vi "Autonomous Independent.vi"() -> ()   [LabVIEW 2023]
doc: "This VI is called when autonomous begins, and will automatically be terminated when autonomous ends. You can carry out timed or sensor driven robot movement independently without needing to return to the caller."
uses:
  <vilib>/Rock Robotics/WPI/SafetyOutput/WPI_SafetyOutputConfigMenu.ctl
  <vilib>/Rock Robotics/WPI/RobotDrive/WPI_RobotDriveDevRef.ctl
  <vilib>/Rock Robotics/WPI/MotorControl/WPI_MotorControlDeviceRef.ctl
  <vilib>/Rock Robotics/WPI/MotorControl/WPI_MotorControlType.ctl
  <vilib>/Rock Robotics/SystemInterfaces/DIO/FPGA_DIOPWMChannel.ctl
  <vilib>/Rock Robotics/WPI/PWM/WPI_PWMDeadband.ctl
  <vilib>/Rock Robotics/SystemInterfaces/DIO/FPGA_DIOChannel.ctl
  <vilib>/Rock Robotics/WPI/ThirdParty/REV Robotics/REVLib/Typedef/Spark MAX Idle Mode.ctl
  <vilib>/Rock Robotics/WPI/Utilities/WPI_GetSetVariantRefNum.vi
  <vilib>/Rock Robotics/Network Tables/NT Read String.vi
  <vilib>/Rock Robotics/Network Tables/NT Write Numeric Array.vi
  <vilib>/Rock Robotics/WPI/ThirdParty/REV Robotics/REVLib/SubVI/Public/SPARK Open Brushed.vi
  <vilib>/Rock Robotics/WPI/ThirdParty/REV Robotics/REVLib/SubVI/Public/SPARK Configure Basic Idle Mode.vi
  <vilib>/Rock Robotics/WPI/ThirdParty/REV Robotics/REVLib/SubVI/Public/SPARK Configure Power Smart Current Limit.vi
  <vilib>/Rock Robotics/WPI/RobotDrive/WPI_RobotDriveArcadeDrive_Standard(NoSaturation).vi
panel:
  out "Current Movement, for debugging":T1 {"Y Joystick Value" scale=1.0..-1.0; "X Joystick Value" scale=-1.0..1.0}
  in  "Array of robot movements":T2(array[cluster])=[{"X Joystick Value"=0.39393939393939403, "Y Joystick Value"=0.0, "Delay (sec)"=1.0, "Movement Name"="turn"}, {"X Joystick Value"=-0.3737373737373737, "Y Joystick Value"=0.0, "Delay (sec)"=1.0, "Movement Name"="turn back"}] {"Y Joystick Value" scale=1.0..-1.0; "X Joystick Value" scale=-1.0..1.0}
  # "Be sure to right-click and choose Data Operations>>Make Current Value default if you want to save the array values with the VI"
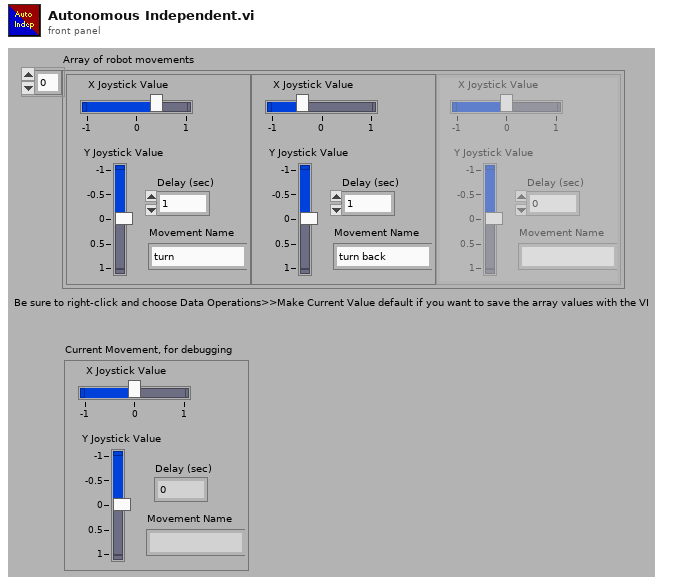
[diagram p1: front panel]
types:
  T1 = cluster{"X Joystick Value":dbl, "Y Joystick Value":dbl, "Delay (sec)":dbl, "Movement Name":string}
  T2 = cluster{"X Joystick Value":dbl, "Y Joystick Value":dbl, "Delay (sec)":dbl, "Movement Name":string}[]
  T3 = typedef "WPI_RobotDriveDevRef.ctl" = cluster{"DevStatus":errorcluster, "Motors[]":T4[], "Square Inputs":bool, "Max Output":dbl}
  T4 = typedef "WPI_MotorControlDeviceRef.ctl" = cluster{"DeviceStatus":errorcluster, "Type":T5, "PWM":cluster{"PWM Channel":T6, "DeadBand":T7}, "CAN":cluster{"Device Number":u8, "SetOutput VI Ref":variant, "GetOutput VI Ref":variant, "Enable VI Ref":variant, "Disable VI Ref":variant, "Data":variant}, "Invert":bool, "DIO PWM":cluster{"PWM \"Enable\" Channel":T6, "DIOChannel":T8, "PWM Rate":dbl}}
  T5 = typedef "WPI_MotorControlType.ctl" = enum16{"PWM", "CAN", "DIO PWM"}
  T6 = typedef "FPGA_DIOPWMChannel.ctl" = enum8{"PWM 0", "PWM 1", "PWM 2", "PWM 3", "PWM 4", "PWM 5", "PWM 6", "PWM 7", "PWM 8", "PWM 9", "PWM MXP 0", "PWM MXP 1", "PWM MXP 2", "PWM MXP 3", "PWM MXP 4", "PWM MXP 5", "PWM MXP 6", "PWM MXP 7", "PWM MXP 8", "PWM MXP 9", "Invalid"}
  T7 = typedef "WPI_PWMDeadband.ctl" = cluster{"Name":string, "maxPositivePwm":i32, "minPositivePwm":i32, "centerPwm":i32, "maxNegativePwm":i32, "minNegativePwm":i32, "angularRange":u16}
  T8 = typedef "FPGA_DIOChannel.ctl" = enum8{"DIO 0", "DIO 1", "DIO 2", "DIO 3", "DIO 4", "DIO 5", "DIO 6", "DIO 7", "DIO 8", "DIO 9", "DIO MXP 0", "DIO MXP 1", "DIO MXP 2", "DIO MXP 3", "DIO MXP 4", "DIO MXP 5", "DIO MXP 6", "DIO MXP 7", "DIO MXP 8", "DIO MXP 9", "DIO MXP 10", "DIO MXP 11", "DIO MXP 12", "DIO MXP 13", "DIO MXP 14", "DIO MXP 15", "SPI Port CS1", "SPI Port CS2", "SPI Port CS3", "SPI Port MISO", "SPI Port MOSI", "Invalid"}
  T9 = typedef "WPI_SafetyOutputConfigMenu.ctl" = enum16{"Enable", "Disable"}
  T10 = typedef "WPI_JoystickDevRef.ctl" = cluster{"Device":T11}
  T11 = typedef "WPI_JoystickDeviceEnum.ctl" = enum16{"USB 0", "USB 1", "USB 2", "USB 3", "USB 4", "USB 5"}
  T12 = typedef "Spark MAX Idle Mode.ctl" = enum16{"Coast", "Brake"}
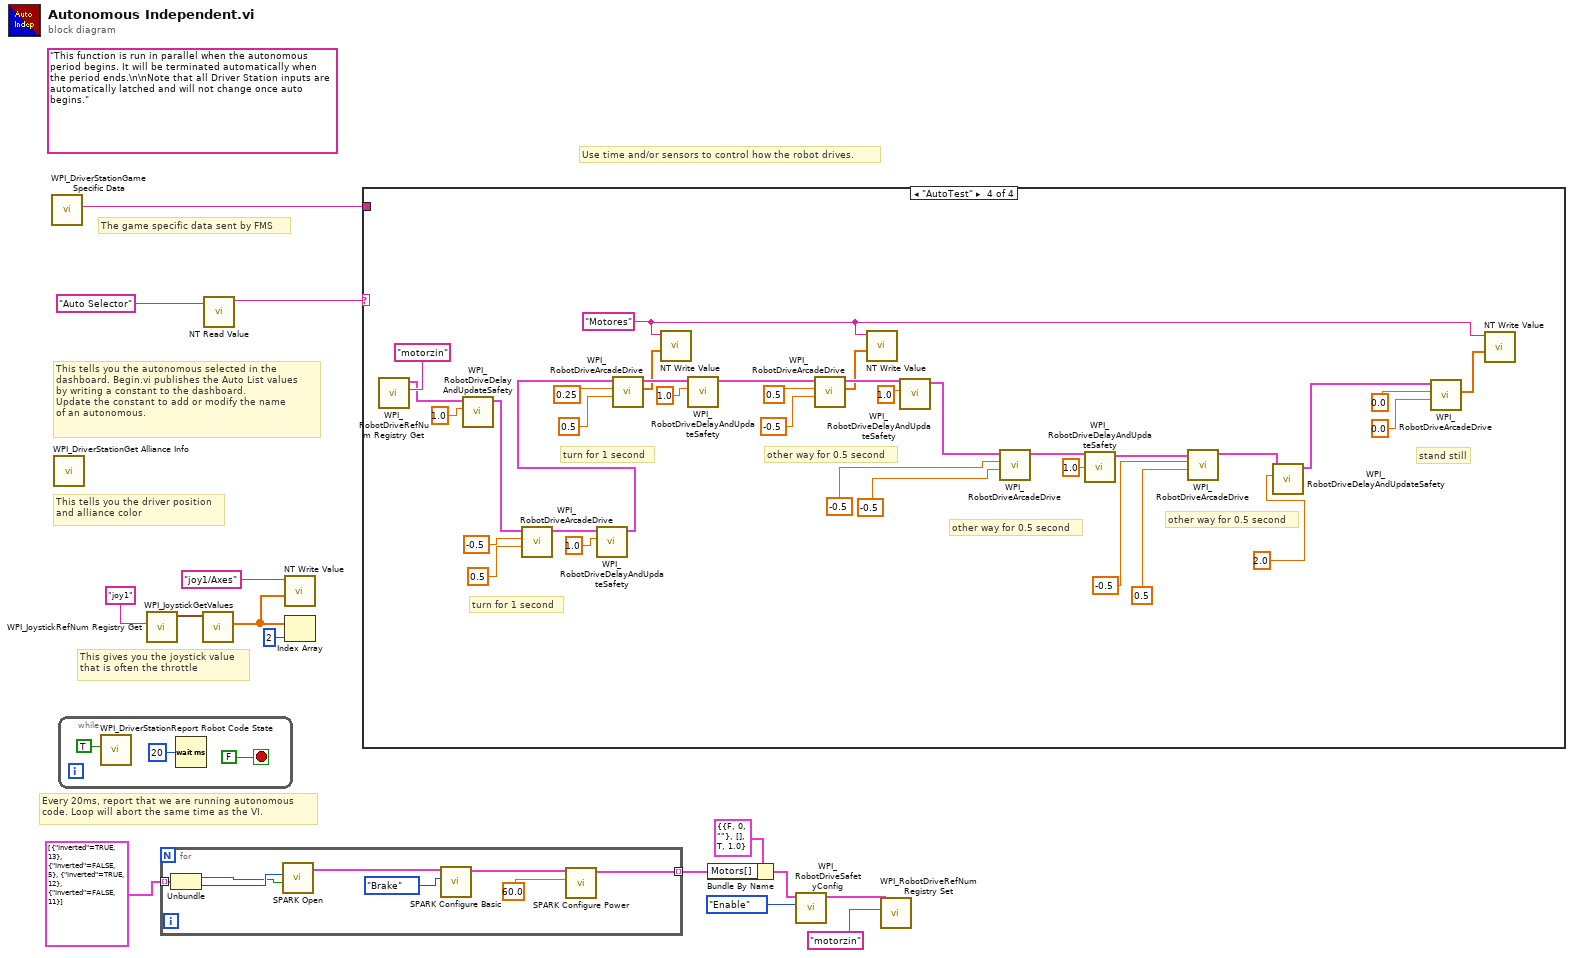
[diagram p0: block diagram]
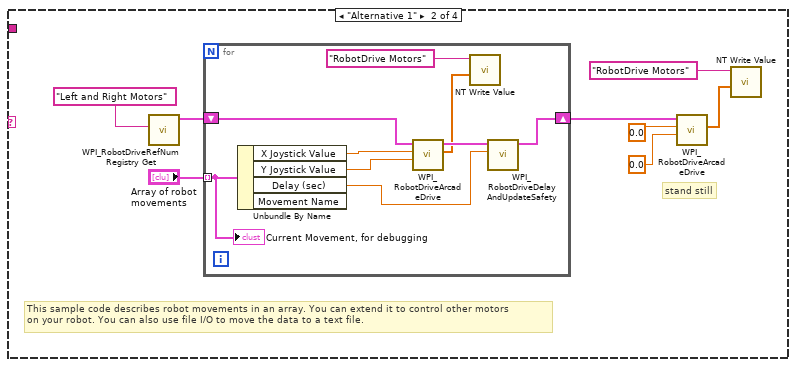
[diagram p3: hidden frame]
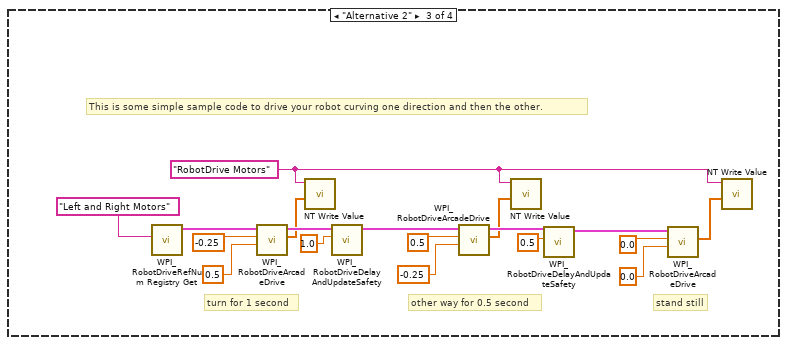
[diagram p4: hidden frame]
diagram:
  (unwired) "This function is run in parallel when the autonomous period begins. It will be terminated automatically when the period ends.\n\nNote that all Driver Station inputs are automatically latched and will not change once auto begins."
  # "The game specific data sent by FMS"
  # "This tells you the autonomous selected in the \ndashboard. Begin.vi publishes the Auto List values\nby writing a constant to the dashboard.\nUpdate the constant to add or modify the name\nof an autonomous."
  # "Every 20ms, report that we are running autonomous\ncode. Loop will abort the same time as the VI."
  # "This gives you the joystick value\nthat is often the throttle"
  # "Use time and/or sensors to control how the robot drives."
  # "This tells you the driver position\nand alliance color"
  n1 = call <vilib>:"WPI_DriverStationGame Specific Data.vi"() -> ("Game Specific Data"=w8:string)  [unwired: 11 in]
  n2 = call <vilib>:"WPI_DriverStationGet Alliance Info.vi"() -> ()  [unwired: 12 out]
  n3 = while {
    stop <- FALSE stop-if-true
    n4 = call <vilib>:"WPI_DriverStationReport Robot Code State.vi"("Autonomous"=TRUE) -> ()  [unwired: 10 in, 1 out]
    n5 = Wait (ms)(milliseconds to wait=u32 20) -> ()  [unwired: 1 out]
  }
  n6 = call <vilib>:"WPI_JoystickRefNum Registry Get.vi"("refnum name"="joy1") -> ("JoystickDevRef"=w14:T10)  [unwired: 1 in, 9 out]
  n7 = for {
    tunnel: cluster{"Inverted":bool, i32}[] [{"Inverted"=TRUE, 13}, {"Inverted"=FALSE, 5}, {"Inverted"=TRUE, 12}, {"Inverted"=FALSE, 11}] ("Array") -> [w26] mode=indexing
    tunnel: [w19] -> w3 mode=indexing
    n8 = Unbundle(w26) -> ("Inverted"=w24:bool, w25:i32)
    n9 = call-poly <vilib>:"SPARK Open.vi"("Invert"=w24, "Device Number"=w25) -> ("MotorControlDeviceRef"=w23:T4)  [unwired: 8 in, 1 out]
    n10 = call-poly <vilib>:"SPARK Configure Basic.vi"("Idle Mode"=Spark_MAX_Idle_Mode."Brake", "MotorControlDeviceRef in"=w23) -> ("MotorControlDeviceRef out"=w22:T4)  [unwired: 8 in, 1 out]
    n11 = call-poly <vilib>:"SPARK Configure Power.vi"("Primay Current Limit (80A)"=60.0, "MotorControlDeviceRef in"=w22) -> ("MotorControlDeviceRef out"=w19:T4)  [unwired: 8 in, 1 out]
  }
  n12 = call <vilib>:"WPI_JoystickGetValues.vi"("JoystickDevRef"=w14) -> ("Axes"=w10:dbl[])  [unwired: 6 in, 4 out]
  n13 = call-poly <vilib>:"NT Read Value.vi"("name"="Auto Selector" ("Name")) -> ("value"=w11:string)  [unwired: 8 in, 2 out]
  n14 = call-poly <vilib>:"NT Write Value.vi"("value"=w10, "name"="joy1/Axes" ("Name")) -> ()  [unwired: 9 in, 1 out]
  n15 = Index Array(array=w10, index=2) -> ()  [unwired: 1 out]
  n16 = case shown="\"AutoTest\"" w11 {
    tunnel: w8 -> [_ _ _ _]
    frame Default {
      # "You can put your main auto here, or you can right-click on the case and make any\nother frame be the default case."
      # "This is the frame that will execute if no selection is made, or if it is not recognized"
    }
    frame "Alternative 1" {
      # "stand still"
      # "This sample code describes robot movements in an array. You can extend it to control other motors\non your robot. You can also use file I/O to move the data to a text file."
      n17 = call <vilib>:"WPI_RobotDriveRefNum Registry Get.vi"("refnum name"="Left and Right Motors") -> ("RobotDriveDevRef"=w33:T3)  [unwired: 1 in, 9 out]
      n18 = for {
        shift-right: [w41] -> w28
        shift-left: w33 -> [w42]
        tunnel: "Array of robot movements" -> [w37] mode=indexing
        n19 = Unbundle By Name(w37) -> ("X Joystick Value"=w40:dbl, "Y Joystick Value"=w39:dbl, "Delay (sec)"=w38:dbl)  [unwired: 1 out]
        n20 = call-poly <vilib>:"WPI_RobotDriveArcadeDrive.vi"("Y axis value"=w39, "X axis value"=w40, "RobotDriveDevRef"=w42) -> ("Motor Values"=w35:dbl[], "RobotDriveDevRef"=w43:T3)  [unwired: 1 in, 6 out]
        n21 = call-poly <vilib>:"NT Write Value.vi"("value"=w35, "name"="RobotDrive Motors" ("Name")) -> ()  [unwired: 9 in, 1 out]
        n22 = call <vilib>:"WPI_RobotDriveDelayAndUpdateSafety.vi"("Delay (s)"=w38, "RobotDriveDevRef"=w43) -> ("RobotDriveDevRef 2"=w41:T3)  [unwired: 8 in, 1 out]
        "Current Movement, for debugging" <- w37
      }
      n23 = call-poly <vilib>:"WPI_RobotDriveArcadeDrive.vi"("Y axis value"=0.0 ("X axis value"), "X axis value"=0.0, "RobotDriveDevRef"=w28) -> ("Motor Values"=w31:dbl[])  [unwired: 1 in, 7 out]
      n24 = call-poly <vilib>:"NT Write Value.vi"("value"=w31, "name"="RobotDrive Motors" ("Name")) -> ()  [unwired: 9 in, 1 out]
    }
    frame "Alternative 2" {
      w45 = "RobotDrive Motors" ("Name")
      # "This is some simple sample code to drive your robot curving one direction and then the other."
      # "stand still"
      # "other way for 0.5 second"
      # "turn for 1 second"
      n25 = call <vilib>:"WPI_RobotDriveRefNum Registry Get.vi"("refnum name"="Left and Right Motors") -> ("RobotDriveDevRef"=w61:T3)  [unwired: 1 in, 9 out]
      n26 = call-poly <vilib>:"WPI_RobotDriveArcadeDrive.vi"("Y axis value"=0.5 ("X axis value"), "X axis value"=-0.25, "RobotDriveDevRef"=w61) -> ("Motor Values"=w44:dbl[], "RobotDriveDevRef"=w54:T3)  [unwired: 1 in, 6 out]
      n27 = call-poly <vilib>:"NT Write Value.vi"("value"=w44, "name"=w45) -> ()  [unwired: 9 in, 1 out]
      n28 = call <vilib>:"WPI_RobotDriveDelayAndUpdateSafety.vi"("Delay (s)"=1.0, "RobotDriveDevRef"=w54) -> ("RobotDriveDevRef 2"=w55:T3)  [unwired: 8 in, 1 out]
      n29 = call-poly <vilib>:"WPI_RobotDriveArcadeDrive.vi"("Y axis value"=-0.25 ("X axis value"), "X axis value"=0.5, "RobotDriveDevRef"=w55) -> ("Motor Values"=w46:dbl[], "RobotDriveDevRef"=w56:T3)  [unwired: 1 in, 6 out]
      n30 = call-poly <vilib>:"NT Write Value.vi"("value"=w46, "name"=w45) -> ()  [unwired: 9 in, 1 out]
      n31 = call <vilib>:"WPI_RobotDriveDelayAndUpdateSafety.vi"("Delay (s)"=0.5, "RobotDriveDevRef"=w56) -> ("RobotDriveDevRef 2"=w57:T3)  [unwired: 8 in, 1 out]
      n32 = call-poly <vilib>:"WPI_RobotDriveArcadeDrive.vi"("Y axis value"=0.0 ("X axis value"), "X axis value"=0.0, "RobotDriveDevRef"=w57) -> ("Motor Values"=w47:dbl[])  [unwired: 1 in, 7 out]
      n33 = call-poly <vilib>:"NT Write Value.vi"("value"=w47, "name"=w45) -> ()  [unwired: 9 in, 1 out]
    }
    frame "AutoTest" {
      w82 = "Motores" ("Name")
      # "turn for 1 second"
      # "other way for 0.5 second"
      # "other way for 0.5 second"
      # "stand still"
      # "other way for 0.5 second"
      # "turn for 1 second"
      n34 = call <vilib>:"WPI_RobotDriveRefNum Registry Get.vi"("refnum name"="motorzin") -> ("RobotDriveDevRef"=w79:T3)  [unwired: 1 in, 9 out]
      n35 = call <vilib>:"WPI_RobotDriveDelayAndUpdateSafety.vi"("Delay (s)"=1.0, "RobotDriveDevRef"=w79) -> ("RobotDriveDevRef 2"=w65:T3)  [unwired: 8 in, 1 out]
      n36 = call-poly <vilib>:"WPI_RobotDriveArcadeDrive.vi"("Y axis value"=0.5 ("X axis value"), "X axis value"=-0.5, "RobotDriveDevRef"=w65) -> ("RobotDriveDevRef"=w63:T3)  [unwired: 1 in, 7 out]
      n37 = call <vilib>:"WPI_RobotDriveDelayAndUpdateSafety.vi"("Delay (s)"=1.0, "RobotDriveDevRef"=w63) -> ("RobotDriveDevRef 2"=w62:T3)  [unwired: 8 in, 1 out]
      n38 = call-poly <vilib>:"WPI_RobotDriveArcadeDrive.vi"("Y axis value"=0.5 ("X axis value"), "X axis value"=0.25, "RobotDriveDevRef"=w62) -> ("Motor Values"=w81:dbl[], "RobotDriveDevRef"=w91:T3)  [unwired: 1 in, 6 out]
      n39 = call-poly <vilib>:"NT Write Value.vi"("value"=w81, "name"=w82) -> ()  [unwired: 9 in, 1 out]
      n40 = call <vilib>:"WPI_RobotDriveDelayAndUpdateSafety.vi"("Delay (s)"=1.0, "RobotDriveDevRef"=w91) -> ("RobotDriveDevRef 2"=w92:T3)  [unwired: 8 in, 1 out]
      n41 = call-poly <vilib>:"WPI_RobotDriveArcadeDrive.vi"("Y axis value"=-0.5 ("X axis value"), "X axis value"=0.5, "RobotDriveDevRef"=w92) -> ("Motor Values"=w83:dbl[], "RobotDriveDevRef"=w93:T3)  [unwired: 1 in, 6 out]
      n42 = call-poly <vilib>:"NT Write Value.vi"("value"=w83, "name"=w82) -> ()  [unwired: 9 in, 1 out]
      n43 = call <vilib>:"WPI_RobotDriveDelayAndUpdateSafety.vi"("Delay (s)"=1.0, "RobotDriveDevRef"=w93) -> ("RobotDriveDevRef 2"=w76:T3)  [unwired: 8 in, 1 out]
      n44 = call-poly <vilib>:"WPI_RobotDriveArcadeDrive.vi"("Y axis value"=-0.5, "X axis value"=-0.5, "RobotDriveDevRef"=w76) -> ("RobotDriveDevRef"=w77:T3)  [unwired: 1 in, 7 out]
      n45 = call <vilib>:"WPI_RobotDriveDelayAndUpdateSafety.vi"("Delay (s)"=1.0, "RobotDriveDevRef"=w77) -> ("RobotDriveDevRef 2"=w73:T3)  [unwired: 8 in, 1 out]
      n46 = call-poly <vilib>:"WPI_RobotDriveArcadeDrive.vi"("Y axis value"=0.5, "X axis value"=-0.5, "RobotDriveDevRef"=w73) -> ("RobotDriveDevRef"=w70:T3)  [unwired: 1 in, 7 out]
      n47 = call <vilib>:"WPI_RobotDriveDelayAndUpdateSafety.vi"("Delay (s)"=2.0, "RobotDriveDevRef"=w70) -> ("RobotDriveDevRef 2"=w69:T3)  [unwired: 8 in, 1 out]
      n48 = call-poly <vilib>:"WPI_RobotDriveArcadeDrive.vi"("Y axis value"=0.0 ("X axis value"), "X axis value"=0.0, "RobotDriveDevRef"=w69) -> ("Motor Values"=w84:dbl[])  [unwired: 1 in, 7 out]
      n49 = call-poly <vilib>:"NT Write Value.vi"("value"=w84, "name"=w82) -> ()  [unwired: 9 in, 1 out]
    }
  }
  n50 = Bundle By Name(cluster=T3 {"DevStatus"={"status"=FALSE, "code"=0, "source"=""}, "Motors[]"=[], "Square Inputs"=TRUE, "Max Output"=1.0} ("RobotDriveDevRef"), "Motors[]"=w3) -> (w6:T3)
  n51 = call <vilib>:"WPI_RobotDriveSafetyConfig.vi"("mode"=WPI_SafetyOutputConfigMenu."Enable", "RobotDriveDevRef"=w6) -> ("RobotDriveDevRef"=w2:T3)  [unwired: 2 in, 7 out]
  n52 = call <vilib>:"WPI_RobotDriveRefNum Registry Set.vi"("refnum name"="motorzin", "RobotDriveDevRef"=w2) -> ()  [unwired: 8 in, 2 out]
